vi "VisualizePodVectors.vi"(10 "Pod Output Vectors":cluster{"Magnitude":dbl, "Direction":dbl}[](array[cluster]), 11 "Picture Ref":refnum<vi>) -> ()   [LabVIEW 2014]
uses:
  Variables/Physical data.vi
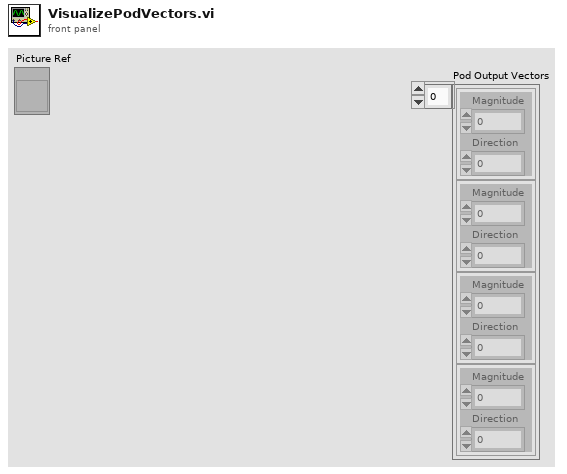
[diagram p1: front panel]
types:
  T1 = typedef "NI_Matrix.lvlib/RealMatrix.ctl" = dbl[][]
  T2 = cluster{"All Pod State Data":cluster{"Drive":cluster{"Drive Motor Output":dbl, "Wheel RPM":dbl, "Linear speed":dbl, "Linear acceleration":dbl, "Encoder Output":dbl, "Vmot":dbl, "Imot":dbl, "Torque":dbl, "Angular Momentum":dbl}, "Turret":cluster{"Turret Motor Output":dbl, "Turret Angle":dbl, "Turret velocity":dbl, "Turret acceleration":dbl, "Encoder Output":dbl, "Vmot":dbl, "Imot":dbl, "Torque":dbl, "Angular Momentum":dbl}, "Pod position (RCS)":cluster{"X":dbl, "Y":dbl, "Z":dbl}}[], "Global Robot Data":cluster{"Position Data":cluster{"Robot Position":cluster{"X":dbl, "Y":dbl, "Z":dbl}, "Robot Velocity":cluster{"X":dbl, "Y":dbl, "Z":dbl}, "Robot Acceleration":cluster{"X":dbl, "Y":dbl, "Z":dbl}}, "Rotation Data":cluster{"Angular Position":cluster{"X":dbl, "Y":dbl, "Z":dbl}, "Angular Velocity":cluster{"X":dbl, "Y":dbl, "Z":dbl}, "Angular Acceleration":cluster{"X":dbl, "Y":dbl, "Z":dbl}}}, "Inertial Characteristics":cluster{"Center of Mass (RCS)":cluster{"X":dbl, "Y":dbl, "Z":dbl}, "Mass Elements":cluster{"X":dbl, "Y":dbl, "Z":dbl, "Mass":dbl, "Name":string}[], "Center of Rotation (RCS)":cluster{"X":dbl, "Y":dbl, "Z":dbl}, "Tensor of Inertia":T1}}
  T3 = cluster{"PodConfigurations":cluster{"Drive":cluster{"Encoder":cluster{"CPft":dbl, "Location":string, "RIO_PinA":i32, "RIO_PinB":i32, "Invert?":bool}, "Motor":cluster{"PID":cluster{"P":dbl, "I":dbl, "D":dbl}, "CANorPWM Channel":i32, "Invert?":bool, "IsCanSRX?":bool, "Output":cluster{"Max":dbl, "Min":dbl}}}, "Turret":cluster{"Encoder":cluster{"ZeroPosVolts":dbl, "Location":string, "RIO_AnalogChannel":i32, "Invert?":bool}, "Motor":cluster{"PID":cluster{"P":dbl, "I":dbl, "D":dbl}, "CANorPWM Channel":i32, "Invert?":bool, "IsCanSRX?":bool, "Output":cluster{"Max":dbl, "Min":dbl}}}, "Misc":cluster{"Pod_Pos":cluster{"X":dbl, "Y":dbl}, "PDP_Channels":cluster{"Drive":i32, "Turret":i32}}}[], "General Configuration":cluster{"Pod Count":i32, "PDP CAN ID":i32, "PCM CAN ID":i32, "BaseRobotMass":dbl}}
  T4 = cluster{"Drive":cluster{"Encoder":cluster{"CPft":dbl, "Location":string, "RIO_PinA":i32, "RIO_PinB":i32, "Invert?":bool}, "Motor":cluster{"PID":cluster{"P":dbl, "I":dbl, "D":dbl}, "CANorPWM Channel":i32, "Invert?":bool, "IsCanSRX?":bool, "Output":cluster{"Max":dbl, "Min":dbl}}}, "Turret":cluster{"Encoder":cluster{"ZeroPosVolts":dbl, "Location":string, "RIO_AnalogChannel":i32, "Invert?":bool}, "Motor":cluster{"PID":cluster{"P":dbl, "I":dbl, "D":dbl}, "CANorPWM Channel":i32, "Invert?":bool, "IsCanSRX?":bool, "Output":cluster{"Max":dbl, "Min":dbl}}}, "Misc":cluster{"Pod_Pos":cluster{"X":dbl, "Y":dbl}, "PDP_Channels":cluster{"Drive":i32, "Turret":i32}}}[]
  T5 = typedef "LVBoundsTypeDef.ctl" = cluster{"Width":u32, "Height":u32}
  T6 = cluster{"Width":u16, "Style":enum32{"Solid", "Dash", "Dot", "DashDot", "DashDotDot"}}
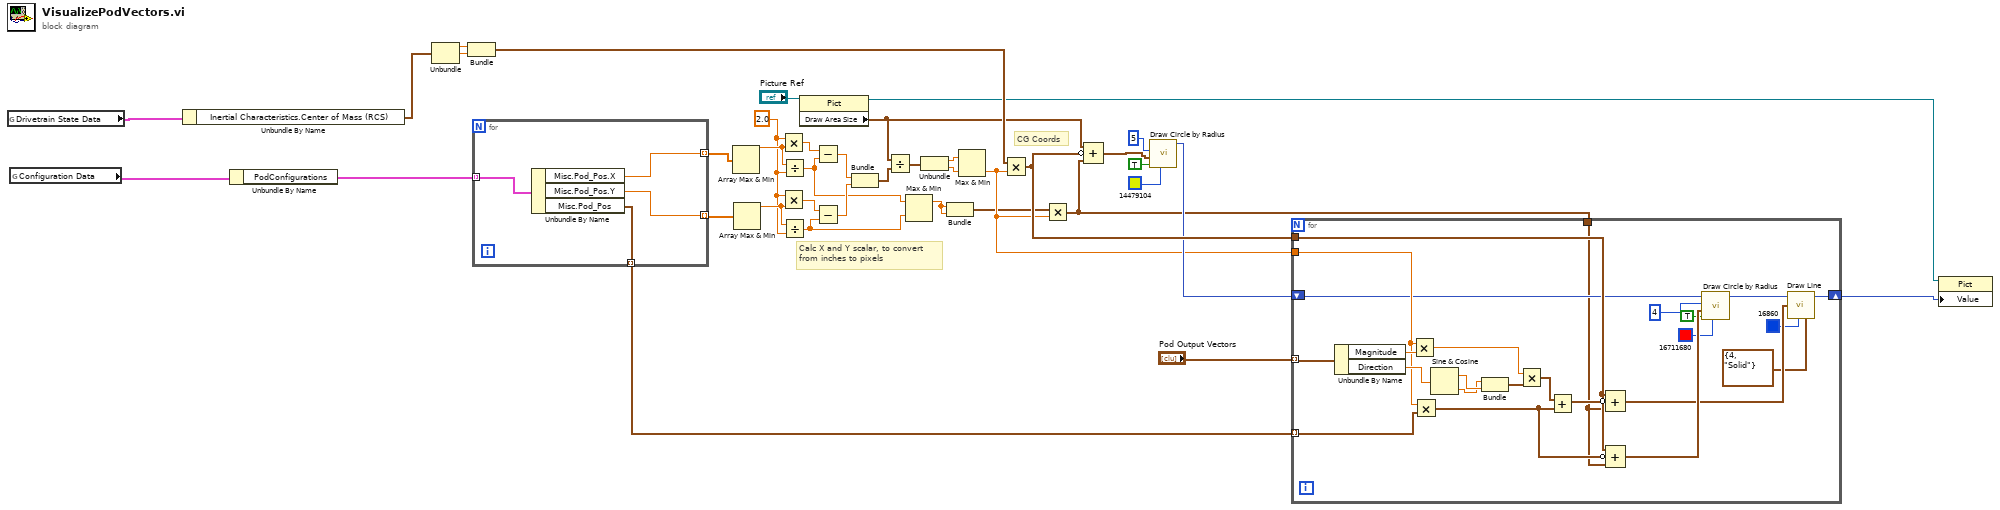
[diagram p0: block diagram]
diagram:
  w30 = 2.0 ("x")
  # "CG Coords"
  # "Calc X and Y scalar, to convert \nfrom inches to pixels"
  n1 = global read "Physical data.vi" "Drivetrain State Data"() -> (w37:T2)
  n2 = global read "Physical data.vi" "Configuration Data"() -> (w36:T3)
  n3 = Unbundle By Name(w37) -> ("Inertial Characteristics.Center of Mass (RCS)"=w27:cluster{"X":dbl, "Y":dbl, "Z":dbl})
  n4 = Unbundle By Name(w36) -> ("PodConfigurations"=w35:T4)
  n5 = Unbundle(w27) -> ("X"=w26:dbl, "Y"=w25:dbl)  [unwired: 1 out]
  n6 = Bundle("X"=w26, "Y"=w25) -> (w24:cluster{"X":dbl, "Y":dbl})  [unwired: 1 in]
  n7 = for {
    tunnel: w35 -> [w42] mode=indexing
    tunnel: [w41] -> w34 mode=indexing
    tunnel: [w40] -> w33 mode=indexing
    tunnel: [w39] -> w16 mode=indexing
    n8 = Unbundle By Name(w42) -> ("Misc.Pod_Pos.X"=w41:dbl, "Misc.Pod_Pos.Y"=w40:dbl, "Misc.Pod_Pos"=w39:cluster{"X":dbl, "Y":dbl})
  }
  n9 = Array Max & Min(array=w34) -> (max value=w32:dbl)  [unwired: 3 out]
  n10 = Array Max & Min(array=w33) -> (max value=w31:dbl)  [unwired: 3 out]
  n11 = Multiply(x=w30, y=w32) -> (x*y=w29:dbl)
  n12 = Multiply(x=w30, y=w31) -> (x*y=w28:dbl)
  n13 = Divide(x=w32, y=w30) -> (x/y=w8:dbl)
  n14 = Divide(x=w31, y=w30) -> (x/y=w7:dbl)
  n15 = property class="Pict"(reference="Picture Ref") -> (reference out=w2:refnum<vi>, "Draw Area Size"=w12:T5)  [unwired: 1 in, 1 out]
  n16 = Subtract(x=w29, y=w8) -> (x-y=w22:dbl)
  n17 = Subtract(x=w28, y=w7) -> (x-y=w21:dbl)
  n18 = Bundle(w22, w21) -> (w20:cluster{dbl, dbl})  [unwired: 1 in]
  n19 = Divide(x=w12, y=w20) -> (x/y=w19:cluster{dbl, dbl})
  n20 = Max & Min(x=w8, y=w7) -> (max(x,y)=w1:dbl)  [unwired: 1 out]
  n21 = Unbundle(w19) -> (w17:dbl, w18:dbl)
  n22 = Bundle(w1, w1) -> (w5:cluster{dbl, dbl})  [unwired: 1 in]
  n23 = Max & Min(x=w17, y=w18) -> (min(x,y)=w6:dbl)  [unwired: 1 out]
  n24 = Multiply(x=w24, y=w6) -> (x*y=w11:cluster{"X":dbl, "Y":dbl})
  n25 = Multiply(x=w5, y=w6) -> (x*y=w4:cluster{dbl, dbl})
  n26 = Compound Arithmetic op=ADD(w12, invert w11, w4) -> (w10:cluster{dbl, dbl})
  n27 = call <vilib>:"Draw Circle by Radius.vi"("color(black)"=u32 14479104, "fill?(F)"=TRUE, "pixel center"=w10, "radius"=i16 5) -> ("new picture"=w9:picture)  [unwired: 7 in]
  n28 = for {
    tunnel: "Pod Output Vectors" -> [w66] mode=indexing
    tunnel: w6 -> [w58]
    tunnel: w16 -> [w57] mode=indexing
    tunnel: w11 -> [w55]
    shift-right: [w50] -> w3
    shift-left: w9 -> [w52]
    tunnel: w4 -> [w43]
    n29 = Unbundle By Name(w66) -> ("Magnitude"=w65:dbl, "Direction"=w64:dbl)
    n30 = Multiply(x=w58, y=w65) -> (x*y=w60:dbl)
    n31 = Multiply(x=w58, y=w57) -> (x*y=w54:cluster{"X":dbl, "Y":dbl})
    n32 = Sine & Cosine(0:w64) -> (1:w63:dbl, 2:w62:dbl)
    n33 = Bundle(w62, w63) -> (w61:cluster{dbl, dbl})  [unwired: 1 in]
    n34 = Multiply(x=w60, y=w61) -> (x*y=w59:cluster{dbl, dbl})
    n35 = Add(x=w59, y=w54) -> (x+y=w56:cluster{dbl, dbl})
    n36 = Compound Arithmetic op=ADD(w55, invert w56, w43) -> (w49:cluster{dbl, dbl})
    n37 = Compound Arithmetic op=ADD(w55, invert w54, w43) -> (w53:cluster{dbl, dbl})
    n38 = call <vilib>:"Draw Circle by Radius.vi"("color(black)"=u32 16711680, "fill?(F)"=TRUE, "pixel center"=w53, "radius"=i16 4, "picture"=w52) -> ("new picture"=w51:picture)  [unwired: 6 in]
    n39 = call <vilib>:"Draw Line.vi"("picture"=w51, "end point"=w49, "color(black)"=u32 16860, "pen"=T6 {"Width"=4, "Style"=enum."Solid"}) -> ("new picture"=w50:picture)  [unwired: 5 in]
  }
  n40 = property class="Pict"(reference=w2, "Value"=w3) -> ()  [unwired: 1 in, 2 out]
